vi "_Read.vi"(8 "error in (no error)":errorcluster, 11 "Std Dev in":refnum<class "Std Dev.lvclass">) -> (0 "error out":errorcluster, 2 "4 Data Points":dbl[](array[numeric]), 3 "Std Dev out":refnum<class "Std Dev.lvclass">)   [LabVIEW 2009, in "Std Dev.lvclass"]
uses:
  Std Dev.lvclass
  Std Dev.lvclass/Std Dev.ctl
  Readable/Readable.lvclass
  <vilib>/Analysis/NI_AALBase.lvlib
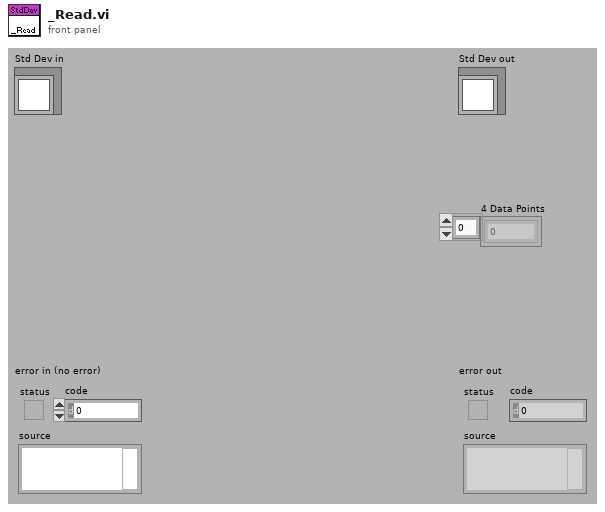
[diagram p1: front panel]
types:
  T1 = typedef "Readable.lvclass/TX Graph.ctl" = cluster{"Data Points":cluster{"t":timestamp, "x":dbl}[]}[]
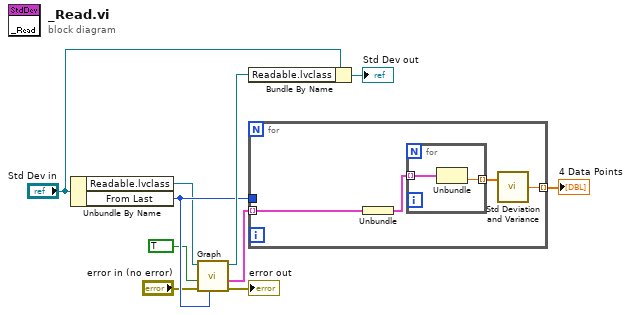
[diagram p0: block diagram]
diagram:
  n1 = Unbundle By Name("Std Dev in") -> ("Readable.lvclass"=w4:refnum<class "Readable.lvclass">, "From Last"=w5:u32)
  n2 = call-dynamic "Graph.vi"("Ring size (points) (1024)"=w5, "error in (no error)"="error in (no error)", "Store Ring? (f)"=TRUE ("Store History? (f)"), "Readable in"=w4) -> ("error out"=→"error out":errorcluster, "Ring Buffers"=w1:T1, "Readable out"=w7:refnum<class "Readable.lvclass">)  [unwired: 1 in, 4 out]
  n3 = Bundle By Name(cluster="Std Dev in", "Readable.lvclass"=w7) -> (→"Std Dev out":refnum<class "Std Dev.lvclass">)
  n4 = for {
    tunnel: [w14] -> w6 mode=indexing
    tunnel: w5 -> [_]
    tunnel: w1 -> [w13] mode=indexing
    n5 = Unbundle(w13) -> ("Data Points"=w12:cluster{"t":timestamp, "x":dbl}[])
    n6 = for {
      tunnel: w12 -> [w16] mode=indexing
      tunnel: [w15] -> w11 mode=indexing
      n7 = Unbundle(w16) -> ("x"=w15:dbl)  [unwired: 1 out]
    }
    n8 = call <vilib>:"Std Deviation and Variance.vi"("X"=w11) -> ("standard deviation"=w14:dbl)  [unwired: 1 in, 2 out]
  }
  "4 Data Points" <- w6
